vi "data claster to array.vi"(11 "Cluster":T1) -> (3 "Array":u64[](array[numeric]))   [LabVIEW 2021]
uses:
  pdw.ctl
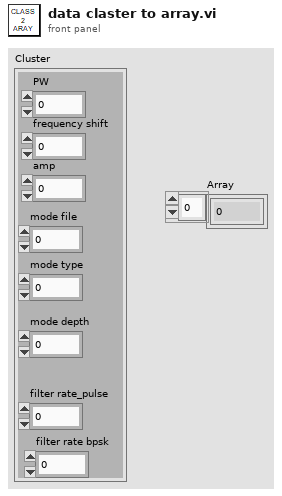
[diagram p1: front panel]
types:
  T1 = typedef "pdw.ctl" = cluster{"PW":u32, "frequency shift":fxp<+/-,48,0>, "amp":fxp<+/-,18,1>, "mode type":u8, "mode file":u8, "mode depth":u32, "filter rate_pulse":u16, "filter rate bpsk":u16}
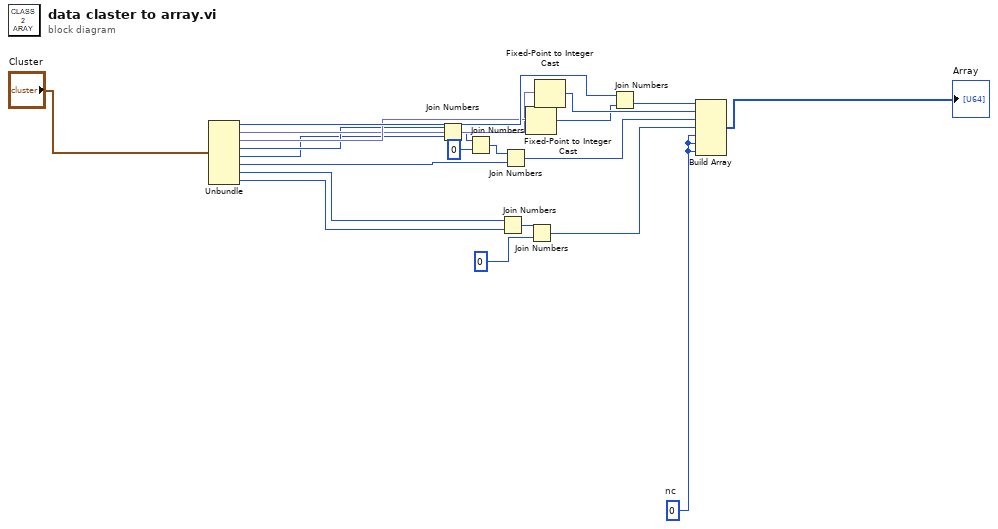
[diagram p0: block diagram]
diagram:
  w2 = u64 0  # nc
  n1 = Unbundle("Cluster") -> ("PW"=w17:u32, "frequency shift"=w15:fxp<+/-,48,0>, "amp"=w16:fxp<+/-,18,1>, "mode type"=w13:u8, "mode file"=w12:u8, "mode depth"=w9:u32, "filter rate_pulse"=w4:u16, "filter rate bpsk"=w3:u16)
  n2 = Join Numbers(hi=w13, lo=w12) -> ((hi.lo)=w11:u16)
  n3 = Join Numbers(hi=w11, lo=u16 0) -> ((hi.lo)=w10:u32)
  n4 = Join Numbers(hi=w4, lo=w3) -> ((hi.lo)=w6:u32)
  n5 = Join Numbers(hi=w10, lo=w9) -> ((hi.lo)=w8:u64)
  n6 = Fixed-Point to Integer Cast(1:w16) -> (0:w18:i32)
  n7 = Join Numbers(hi=w6, lo=u32 0) -> ((hi.lo)=w5:u64)
  n8 = Fixed-Point to Integer Cast(1:w15) -> (0:w20:i64)
  n9 = Join Numbers(hi=w17, lo=w18) -> ((hi.lo)=w19:u64)
  n10 = Build Array(w19, w20, w8, w5, w2, w2, w2) -> (→"Array":u64[])
